vi "vi ondas.vi"() -> ()   [LabVIEW 2018]
uses:
  <vilib>/Utility/file.llb/Read Delimited Spreadsheet (string).vi
  <vilib>/Analysis/NI_AALPro.lvlib
panel:
  out "String 2":string
  out "String":string
  in  "dt (s)":dbl=0.001 format="%#_13g"
  out "Forma de Onda":cluster{dbl[], "Amp Spectrum Mag (Vrms)":dbl[]}(graph)
  out "Magnitude":cluster{dbl[], "Amp Spectrum Mag (Vrms)":dbl[]}(graph)
  out "df (Hz)":dbl format="%0.2f"
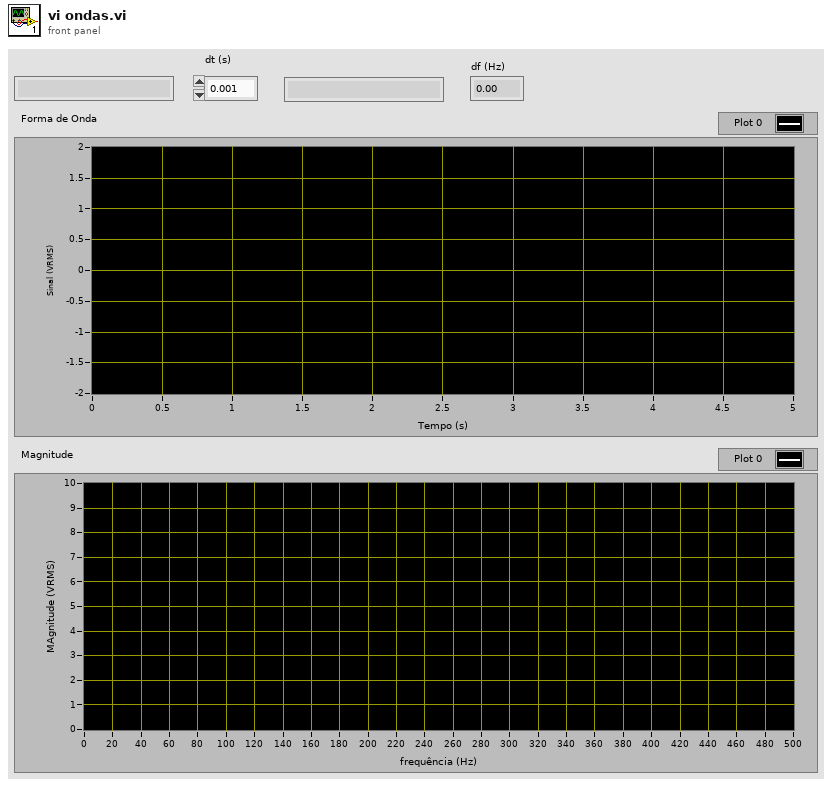
[diagram p1: front panel]
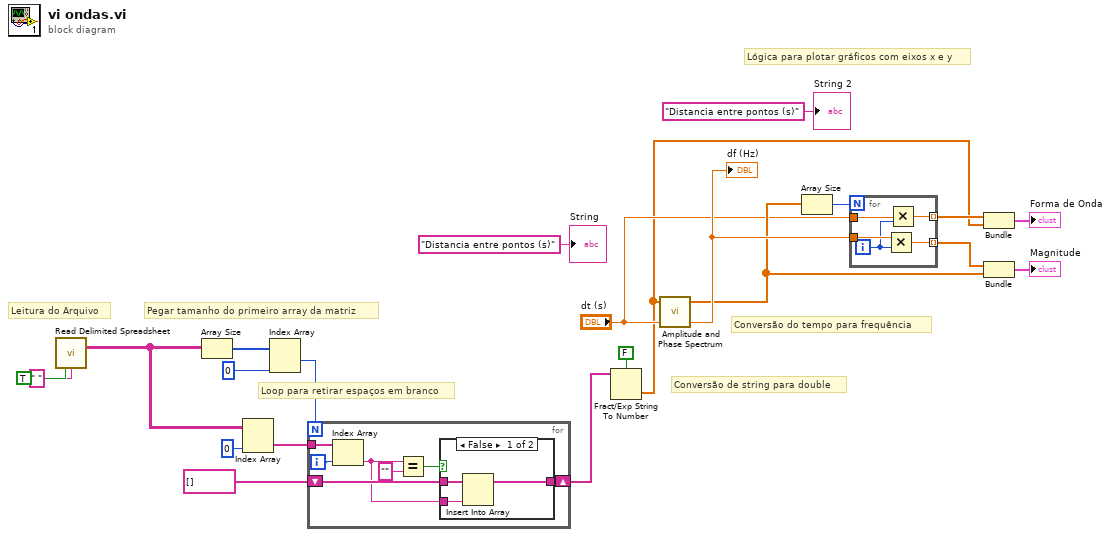
[diagram p0: block diagram]
diagram:
  # "Conversão do tempo para frequência"
  # "Lógica para plotar gráficos com eixos x e y"
  # "Conversão de string para double"
  # "Loop para retirar espaços em branco"
  # "Pegar tamanho do primeiro array da matriz"
  # "Leitura do Arquivo"
  n1 = call-poly <vilib>:"Read Delimited Spreadsheet.vi"("transpose? (F)"=TRUE, "delimiter (\\t)"=" " ("delimiter (\\t)")) -> ("all rows"=w3:string[][])  [unwired: 8 in, 5 out]
  n2 = Array Size(array=w3) -> (size(s)=w21:i32[])
  n3 = Index Array "Index Array"(array=w3, index (col)=0 ("disabled index (col)")) -> (element=w18:string[])  [unwired: 1 in]
  n4 = Index Array "Index Array"(array=w21, index #1=0 ("index")) -> (element #1=w19:i32)  [unwired: 1 in, 1 out]
  n5 = for {
    N: w19 -> [_]
    tunnel: w18 -> [w28]
    shift-right: [w26] -> w16
    shift-left: string[] [] -> [w25]
    i -> [w23]
    n6 = Index Array "Index Array"(array=w28, index=w23) -> (element=w24:string)
    n7 = Equal?(x=w24, y="" ("delimiter (\\t)")) -> (x = y?=w27:bool)
    n8 = case shown="False" w27 {
      tunnel: w24 -> [w32 _]
      tunnel: [w31 w33] -> w26
      tunnel: w25 -> [w30 w33]
      frame False {
        n9 = Insert Into Array "Insert Into Array"(array=w30, new element=w32) -> (w31:string[])  [unwired: 1 in]
      }
      frame True {
      }
    }
  }
  n10 = Fract/Exp String To Number(use system decimal point (T)=FALSE, string=w16) -> (number=w6:dbl[])  [unwired: 2 in, 1 out]
  n11 = call <vilib>:"Amplitude and Phase Spectrum.vi"("dt"="dt (s)", "Signal (V)"=w6) -> ("df"=w13:dbl, "Amp Spectrum Mag (Vrms)"=w12:dbl[])  [unwired: 1 in, 1 out]
  "df (Hz)" <- w13
  n12 = Array Size(array=w12) -> (size(s)=w14:i32)
  n13 = for {
    N: w14 -> [_]
    tunnel: w13 -> [w38]
    tunnel: [w37] -> w7 mode=indexing
    tunnel: "dt (s)" -> [w36]
    tunnel: [w34] -> w9 mode=indexing
    i -> [w35]
    n14 = Multiply(x=w38, y=w35) -> (x*y=w37:dbl)
    n15 = Multiply(x=w36, y=w35) -> (x*y=w34:dbl)
  }
  n16 = Bundle(w9, w6) -> (→"Forma de Onda":cluster{dbl[], dbl[]})  [unwired: 1 in]
  n17 = Bundle(w7, "Amp Spectrum Mag (Vrms)"=w12) -> (→"Magnitude":cluster{dbl[], "Amp Spectrum Mag (Vrms)":dbl[]})  [unwired: 1 in]
  "String" <- "Distancia entre pontos (s)" ("String")
  "String 2" <- "Distancia entre pontos (s)" ("String")
